vi "ReadTriggerChannelNode.vi"(8 "Error In":errorcluster, 11 "Multiplexer Node In":refnum<k20>) -> (0 "Error Out":errorcluster, 2 "Trigger Channel Configuration":T1, 3 "Multiplexer Node Out":refnum<k20>)   [LabVIEW 2012]
uses:
  TriggerChannelConfiguration.ctl
  driver/Public/Controls/TriggerSource.ctl
  <vilib>/xml/NI_XML.lvlib
  driver/Keithley-7001.lvlib
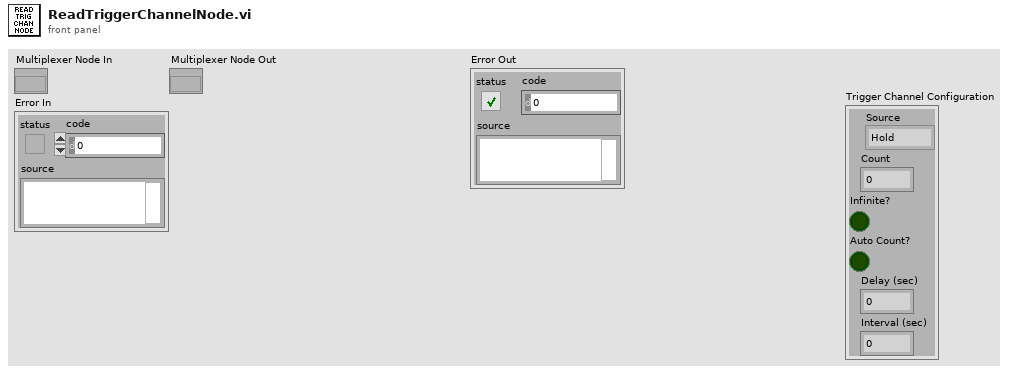
[diagram p1: front panel]
types:
  T1 = typedef "TriggerChannelConfiguration.ctl" = cluster{"Source":T2, "Count":u32, "Infinite?":bool, "Auto Count?":bool, "Delay (sec)":dbl, "Interval (sec)":dbl}
  T2 = typedef "Keithley-7001.lvlib/TriggerSource.ctl" = enum16{"Hold", "Immediate", "Manual", "Bus", "TLink", "External", "Timer"}
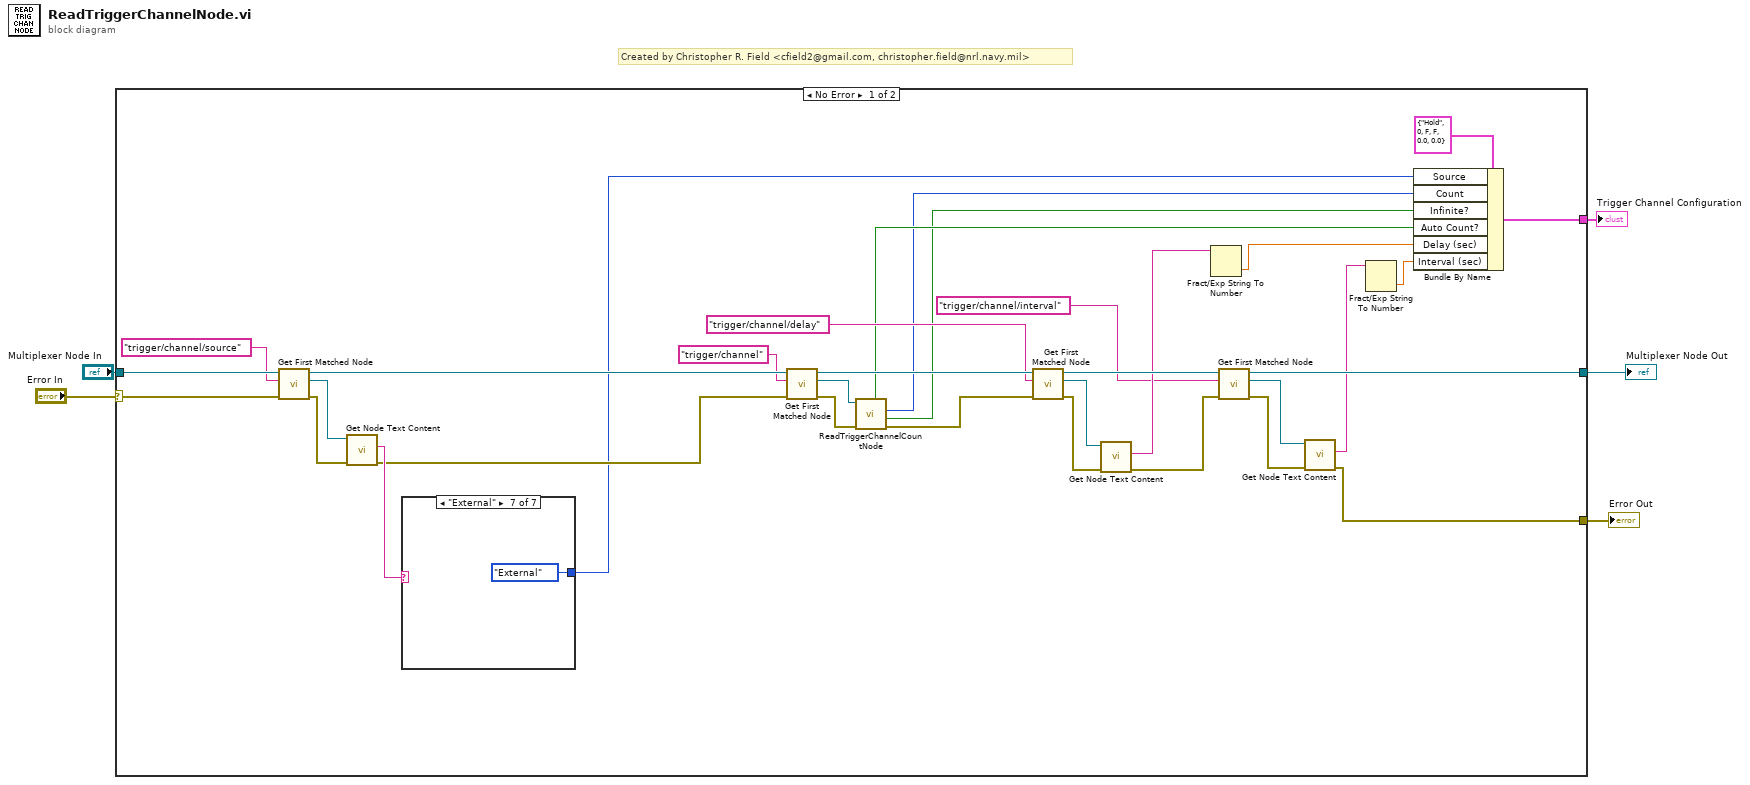
[diagram p0: block diagram]
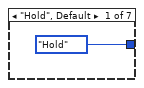
[diagram p2: hidden frame]
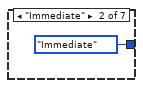
[diagram p3: hidden frame]
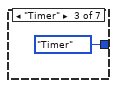
[diagram p4: hidden frame]
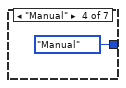
[diagram p5: hidden frame]
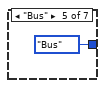
[diagram p6: hidden frame]
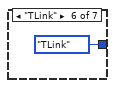
[diagram p7: hidden frame]
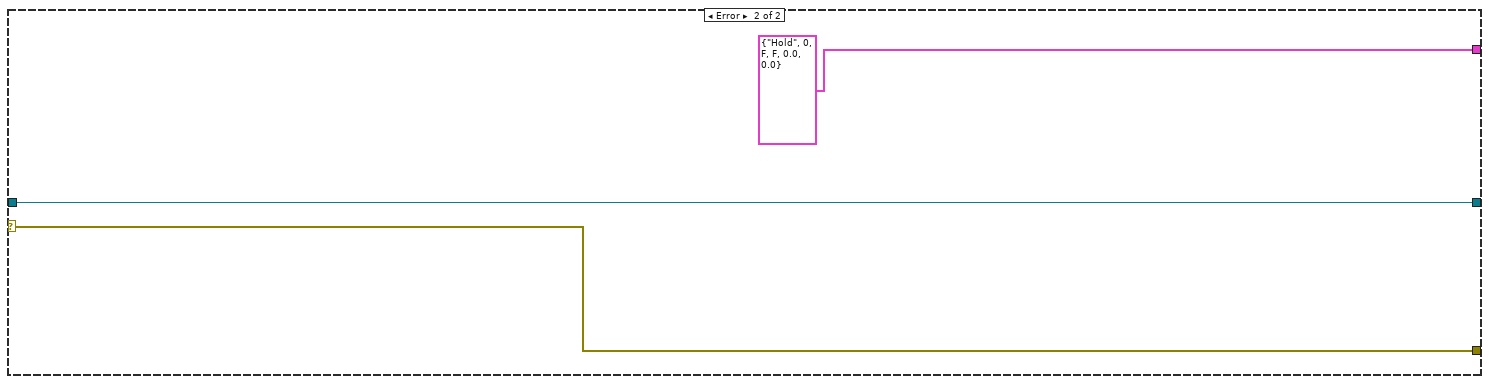
[diagram p8: hidden frame]
diagram:
  # "Created by Christopher R. Field <cfield2@gmail.com, christopher.field@nrl.navy.mil>"
  n1 = case shown="No Error" "Error In" {
    selector: "Error In" -> [w34 w47]
    tunnel: "Multiplexer Node In" -> [w38 w48]
    tunnel: [w20 w47] -> w3
    tunnel: [w24 w48] -> w2
    tunnel: [w13 T1 {"Source"=enum."Hold", "Count"=0, "Infinite?"=FALSE, "Auto Count?"=FALSE, "Delay (sec)"=0.0, "Interval (sec)"=0.0} ("Trigger Channel Configuration")] -> w1
    frame No Error {
      n2 = call <vilib>:"Get First Matched Node.vi"("error in (no error)"=w34, "XPath expression"="trigger/channel/source", "node in"=w38) -> ("error out"=w35:errorcluster, "node result"=w36:refnum<k20>, "node out"=w32:refnum<k20>)  [unwired: 6 in]
      n3 = call <vilib>:"Get Node Text Content.vi"("error in (no error)"=w35, "node in"=w36) -> ("error out"=w30:errorcluster, "node text"=w33:string)  [unwired: 7 in, 1 out]
      n4 = case shown="\"External\"" w33 {
        tunnel: [TriggerSource."Hold" ("Source") TriggerSource."Immediate" ("Source") TriggerSource."Timer" ("Source") TriggerSource."Manual" ("Source") TriggerSource."Bus" ("Source") TriggerSource."TLink" ("Source") TriggerSource."External" ("Source")] -> w12
        frame "Hold", Default {
        }
        frame "Immediate" {
        }
        frame "Timer" {
        }
        frame "Manual" {
        }
        frame "Bus" {
        }
        frame "TLink" {
        }
        frame "External" {
        }
      }
      n5 = call <vilib>:"Get First Matched Node.vi"("error in (no error)"=w30, "XPath expression"="trigger/channel", "node in"=w32) -> ("error out"=w7:errorcluster, "node result"=w11:refnum<k20>, "node out"=w29:refnum<k20>)  [unwired: 6 in]
      n6 = call "ReadTriggerChannelCountNode.vi"("Error In"=w7, "Trigger Node In"=w11) -> ("Error Out"=w6:errorcluster, "Infinite?"=w8:bool, "Count"=w9:u32, "Auto?"=w10:bool)  [unwired: 5 in, 1 out]
      n7 = call <vilib>:"Get First Matched Node.vi"("error in (no error)"=w6, "XPath expression"="trigger/channel/delay", "node in"=w29) -> ("error out"=w26:errorcluster, "node result"=w27:refnum<k20>, "node out"=w25:refnum<k20>)  [unwired: 6 in]
      n8 = call <vilib>:"Get Node Text Content.vi"("error in (no error)"=w26, "node in"=w27) -> ("error out"=w23:errorcluster, "node text"=w19:string)  [unwired: 7 in, 1 out]
      n9 = Fract/Exp String To Number(string=w19) -> (number=w18:dbl)  [unwired: 3 in, 1 out]
      n10 = call <vilib>:"Get First Matched Node.vi"("error in (no error)"=w23, "XPath expression"="trigger/channel/interval", "node in"=w25) -> ("error out"=w21:errorcluster, "node result"=w22:refnum<k20>, "node out"=w24:refnum<k20>)  [unwired: 6 in]
      n11 = call <vilib>:"Get Node Text Content.vi"("error in (no error)"=w21, "node in"=w22) -> ("error out"=w20:errorcluster, "node text"=w17:string)  [unwired: 7 in, 1 out]
      n12 = Fract/Exp String To Number(string=w17) -> (number=w16:dbl)  [unwired: 3 in, 1 out]
      n13 = Bundle By Name(cluster=T1 {"Source"=enum."Hold", "Count"=0, "Infinite?"=FALSE, "Auto Count?"=FALSE, "Delay (sec)"=0.0, "Interval (sec)"=0.0} ("Trigger Channel Configuration"), "Source"=w12, "Count"=w9, "Infinite?"=w8, "Auto Count?"=w10, "Delay (sec)"=w18, "Interval (sec)"=w16) -> (w13:T1)
    }
    frame Error {
    }
  }
  "Error Out" <- w3
  "Multiplexer Node Out" <- w2
  "Trigger Channel Configuration" <- w1
